vi "main.vi"   [LabVIEW 2023]
types:
  T1 = enum32{"Invalid", "Standard", "Closed", "Hidden", "Minimized", "Maximized"}
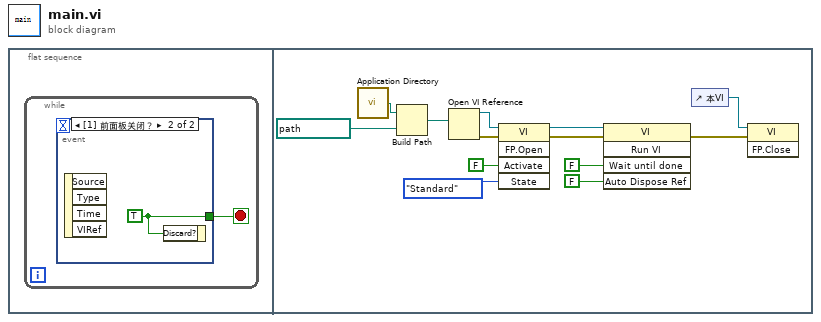
[diagram p0: block diagram]
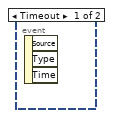
[diagram p2: hidden frame]
diagram:
  n1 = flat-sequence {
    frame #0 {
      n2 = while {
        stop <- w1 stop-if-true
        n3 = event shown="[1] 前面板关闭？" {
          selector: _ -> [_ _]
          dyn-events: _ -> [_ _]
          timeout: _ -> [_ _]
          tunnel: [_ w2] -> w1
          event Timeout {
            n4 = event-data() -> ()  [unwired: 1 in, 3 out]
          }
          event Panel Close? {
            w2 = TRUE ("放弃？")
            n5 = event-data() -> ()  [unwired: 1 in, 4 out]
            n6 = event-data("Discard?"=w2) -> ()  [unwired: 1 in, 1 out]
          }
        }
      }
    }
    frame #1 {
      n7 = call <vilib>:"Application Directory.vi"() -> ("Application Directory"=w14:path)
      n8 = Build Path(base path=w14, name or relative path=path "登录界面.vi" ("名称或相对路径")) -> (appended path=w12:path)
      n9 = Open VI Reference(vi path=w12) -> (vi reference=w11:refnum<vi>, error out=w4:errorcluster)  [unwired: 5 in]
      n10 = invoke class="VI" method="FP.Open"(reference=w11, error in=w4, "Activate"=FALSE ("激活？"), "State"=T1."Standard" ("状态")) -> (reference out=w8:refnum<vi>, error out=w5:errorcluster)  [unwired: 1 in, 3 out]
      n11 = invoke class="VI" method="Run VI"(reference=w8, error in=w5, "Wait until done"=FALSE ("结束前等待"), "Auto Dispose Ref"=FALSE ("自动销毁引用")) -> (error out=w3:errorcluster)  [unwired: 1 in, 4 out]
      n12 = control-ref of="本VI"() -> (w15:refnum<vi>)
      n13 = invoke class="VI" method="FP.Close"(reference=w15, error in=w3) -> ()  [unwired: 1 in, 3 out]
    }
  }
